vi "Configure USIM.vi"(6 "MSIN (\"\")":string, 7 "MNC (\"\")":string, 8 "error in (no error)":errorcluster, 9 "MCC (\"\")":string, 10 "SIM Profile Name (\"\")":string, 11 "VISA resource name":refnum<visa-resource-name>) -> (0 "error out":errorcluster, 3 "VISA resource name out":refnum<visa-resource-name>)   [LabVIEW 2020, in "Rohde&Schwarz CMXP Base.lvlib"]
doc: "The universal subscriber identity module (USIM) contains the international mobile subscriber identity (IMSI) and security parameters for authentication and ciphering in the mobile network.\n\nAttributes:\nRSCMXPBASE_ATTR_USIM_MOBILE_COUNTRY_CODE\nRSCMXPBASE_ATTR_USIM_MOBILE_NETWORK_CODE\nRSCMXPBASE_ATTR_USIM_MOBILE_SUBSCRIBER_IDENTIFICATION_NUMBER\n\nRemote-control commands:\n[CONFigure:]SIMProfile:USIM:MCC\n[CONFigure:]SIMProfile:USIM:MNC\n[CONFigure:]SIMProfile:USIM:MSIN"
uses:
  <instrlib>/Rohde&Schwarz CMXP Base/Rohde&Schwarz CMXP Base.lvlib
  <instrlib>/Rohde&Schwarz CMXP Base/Private/rsidr_core.llb/rsidr_core.lvlib
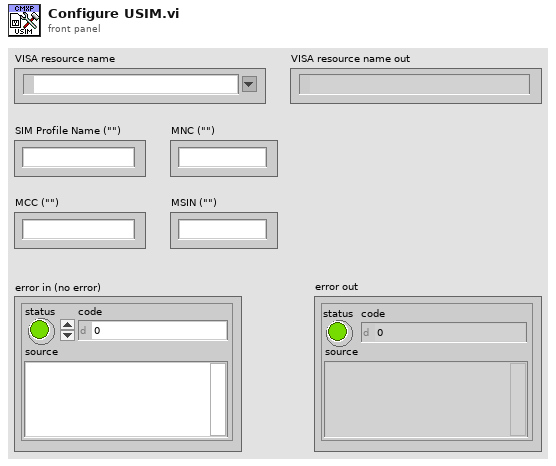
[diagram p1: front panel]
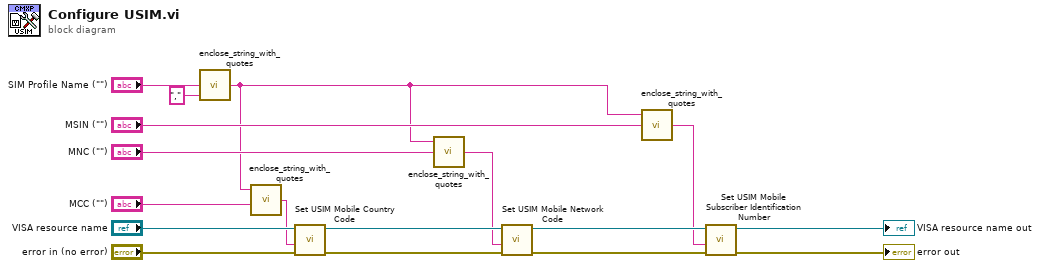
[diagram p0: block diagram]
diagram:
  n1 = call <instrlib>:"enclose_string_with_quotes.vi"("String after"=",", "String to enclose"="SIM Profile Name (\"\")") -> ("String out"=w1:string)  [unwired: 3 in]
  n2 = call <instrlib>:"enclose_string_with_quotes.vi"("String to enclose"="MCC (\"\")", "String before"=w1) -> ("String out"=w4:string)  [unwired: 3 in]
  n3 = call "Set USIM Mobile Country Code"("error in (no error)"="error in (no error)", "USIM Mobile Country Code ()"=w4, "instrument handle"="VISA resource name") -> ("error out"=w15:errorcluster, "instrument handle out"=w14:refnum<visa-resource-name>)  [unwired: 7 in]
  n4 = call <instrlib>:"enclose_string_with_quotes.vi"("String to enclose"="MNC (\"\")", "String before"=w1) -> ("String out"=w6:string)  [unwired: 3 in]
  n5 = call "Set USIM Mobile Network Code"("error in (no error)"=w15, "USIM Mobile Network Code ()"=w6, "instrument handle"=w14) -> ("error out"=w13:errorcluster, "instrument handle out"=w12:refnum<visa-resource-name>)  [unwired: 7 in]
  n6 = call <instrlib>:"enclose_string_with_quotes.vi"("String to enclose"="MSIN (\"\")", "String before"=w1) -> ("String out"=w2:string)  [unwired: 3 in]
  n7 = call "Set USIM Mobile Subscriber Identification Number"("error in (no error)"=w13, "USIM Mobile Subscriber Identification Number ()"=w2, "instrument handle"=w12) -> ("error out"=→"error out":errorcluster, "instrument handle out"=→"VISA resource name out":refnum<visa-resource-name>)  [unwired: 7 in]
